vi "Simple Post Build Generate Arduino Code Template for User Projects.vi"(5 "Files Generated by Build":path[](array[path]), 6 "Top Level/Always Included VIs":path[](array[path]), 7 "Destination Path":path, 8 "error in (no error)":errorcluster, 9 "Target Name":string, 10 "Build Specification Name":string, 11 "Project Path":path) -> (0 "error out":errorcluster)   [LabVIEW 2018]
doc: "Simple template to show user how to use post build action in build specification to automatize transcript process.\nAll what's needed to do with this VI is copy it to your project and set it as post-build action.\n\nThis will transcript just first \"always include\" VI."
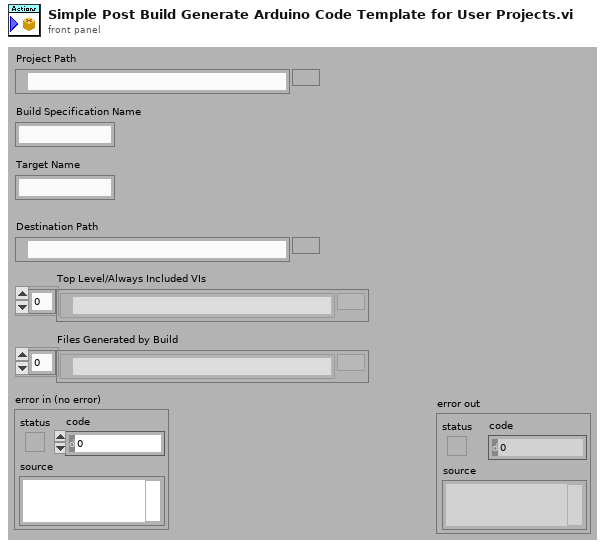
[diagram p1: front panel]
types:
  T1 = enum16{"open", "replace", "create", "open or create", "replace or create", "replace or create with confirmation"}
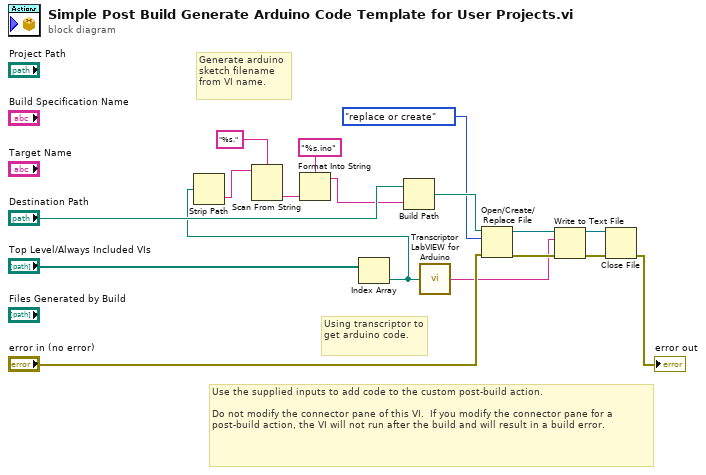
[diagram p0: block diagram]
diagram:
  # "Generate arduino sketch filename from VI name."
  # "Using transcriptor to get arduino code."
  # "Use the supplied inputs to add code to the custom post-build action.\n\nDo not modify the connector pane of this VI.  If you modify the connector pane for a post-build action, the VI will not run after the build and will result in a build error."
  n1 = Index Array(array="Top Level/Always Included VIs") -> (element=w6:path)  [unwired: 1 in]
  n2 = Strip Path(path=w6) -> (name=w5:string)  [unwired: 1 out]
  n3 = Scan From String(format string="%s.", input string=w5) -> (output 1=w2:string)  [unwired: 3 in, 3 out]
  n4 = Format Into String(format string="%s.ino", w2) -> (resulting string=w1:string)  [unwired: 2 in, 1 out]
  n5 = Build Path(base path="Destination Path", name or relative path=w1) -> (appended path=w16:path)
  n6 = call "Transcriptor LabVIEW for Arduino.vi"("vi path"=w6) -> ("transcripted code"=w7:string)
  n7 = Open/Create/Replace File(file path (use dialog)=w16, error in="error in (no error)", operation (0:open)=T1."replace or create") -> (refnum out=w14:refnum<file>, error out=w15:errorcluster)  [unwired: 3 in, 1 out]
  n8 = Write to Text File(file (use dialog)=w14, text=w7, error in=w15) -> (refnum out=w11:refnum<file>, error out=w12:errorcluster)  [unwired: 1 in, 1 out]
  n9 = Close File(refnum=w11, error in=w12) -> (error out=→"error out":errorcluster)  [unwired: 1 out]
